vi "PI Organize Prompt Parameters.vi"(10 "Prompt Measurement Test Parameters":T6, 11 "Results":T1={"Measurement Cycles"=0, "Response"="", "Measurement"={"sxFieldId"="", "sValue"="", "nDataType"=enum."Scalar", "sUnits"="", "sDisplayName"=""}, "Limit"={"Limits On"=TRUE, "Limits"=[]}, "Status Array"=[]}) -> (3 "Results out":T1={"Measurement Cycles"=0, "Response"="", "Measurement"={"sxFieldId"="", "sValue"="", "nDataType"=enum."Scalar", "sUnits"="", "sDisplayName"=""}, "Limit"={"Limits On"=TRUE, "Limits"=[]}, "Status Array"=[]})   [LabVIEW 2011]
uses:
  TypeDefs/PI Test Parameters.ctl
  TypeDefs/PI Measurement Cluster.ctl
  TypeDefs/PI Limit Parameters.ctl
  TypeDefs/PI Limit Definition.ctl
  TypeDefs/PI Limit Comparison.ctl
  TypeDefs/PI Results.ctl
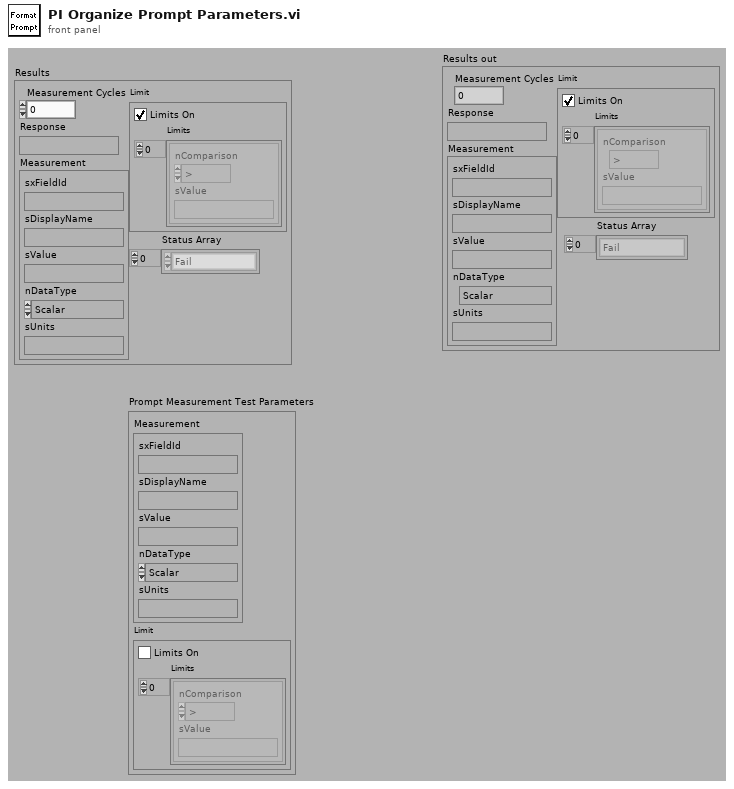
[diagram p1: front panel]
types:
  T1 = typedef "PI Results.ctl" = cluster{"Measurement Cycles":i32, "Response":string, "Measurement":T2, "Limit":T3, "Status Array":enum16{"Fail", "Pass", "Abort", "Error", "Done", "Pass by Sample", "Fail by Sample", "Pass Override", "Fail Override", "Not Tested"}[]}
  T2 = typedef "PI Measurement Cluster.ctl" = cluster{"sxFieldId":string, "sValue":string, "nDataType":enum16{"Scalar", "Enumeration"}, "sUnits":string, "sDisplayName":string}
  T3 = typedef "PI Limit Parameters.ctl" = cluster{"Limits On":bool, "Limits":T4[]}
  T4 = typedef "PI Limit Definition.ctl" = cluster{"nComparison":T5, "sValue":string}
  T5 = typedef "PI Limit Comparison.ctl" = enum16{">", ">=", "<", "<=", "<>", "="}
  T6 = typedef "PI Test Parameters.ctl" = cluster{"Measurement":T2, "Limit":T3}
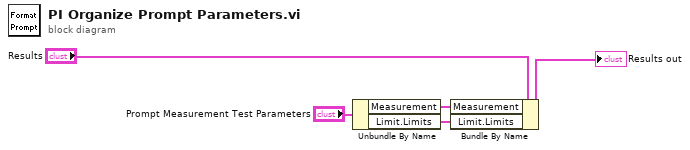
[diagram p0: block diagram]
diagram:
  n1 = Unbundle By Name("Prompt Measurement Test Parameters") -> ("Measurement"=w2:T2, "Limit.Limits"=w1:T4[])
  n2 = Bundle By Name(cluster="Results", "Measurement"=w2, "Limit.Limits"=w1) -> (→"Results out":T1)
